vi "校准设置页.vi"() -> ()   [LabVIEW 2016, in "斯坦道通用流路CODmn.lvlib"]
uses:
  <vilib>/regexp/Match Regular Expression.xnode
  <vilib>/ptbypt/NI_PtbyPt.lvlib
panel:
  in  "校准任务":bool
  in  "历史数据导入":T1(radio)
  out "刷新时间":string
  out "模型刷新":bool
  in  "校准按钮":T1(radio)
  in  "仪器写入":bool
  in  "辅助计算":bool
  in  "曲线模型":T2={"标液浓度1"=0.0, "测量吸光度1"=0.0, "样品1启用"=FALSE, "标液浓度2"=0.0, "测量吸光度2"=0.0, "样品2启用"=FALSE, "标液浓度3"=0.0, "测量吸光度3"=0.0, "样品3启用"=FALSE, "标液浓度4"=0.0, "测量吸光度4"=0.0, "样品4启用"=FALSE, "标液浓度5"=0.0, "测量吸光度5"=0.0, "样品5启用"=FALSE, "模型"=enum."线性", "精度"=4.0, "XY图"=[], "拟合公式"="", "r^2"=0.0, "标样一校准时间"=timestamp(0 s since 1904-01-01), "标样二校准时间"=timestamp(0 s since 1904-01-01), "标样三校准时间"=timestamp(0 s since 1904-01-01), "标样四校准时间"=timestamp(0 s since 1904-01-01), "标样五校准时间"=timestamp(0 s since 1904-01-01), "二次方程"={"c"=0.0, "x"=0.0, "x^2"=0.0}, "标定时间"=timestamp(0 s since 1904-01-01)} {"标定时间" format="%<%y/%m/%d %H:%M:%S>T"; "标样五校准时间" format="%<%y/%m/%d %H:%M:%S>T"; "标样四校准时间" format="%<%y/%m/%d %H:%M:%S>T"; "标样三校准时间" format="%<%y/%m/%d %H:%M:%S>T"; "标样二校准时间" format="%<%y/%m/%d %H:%M:%S>T"; "标样一校准时间" format="%<%y/%m/%d %H:%M:%S>T"; "r^2" format="%.7f"; "测量吸光度5" format="%#.6f"; "测量吸光度4" format="%#.6f"; "测量吸光度3" format="%#.6f"; "测量吸光度2" format="%#.6f"; "测量吸光度1" format="%#.6f"}
  in  "测量模式":T3(ring)
  in  "参数下拉列表":u16(ring) items=["氨氮"=3]
  in  "量程下拉列表":enum16{"低量程", "高量程"}(ring)
  # "校准时间"
  # "标液浓度"
  # "吸光值"
  # "标样一"
  # "标样二"
  # "标样三"
  # "零点"
  # "跨度"
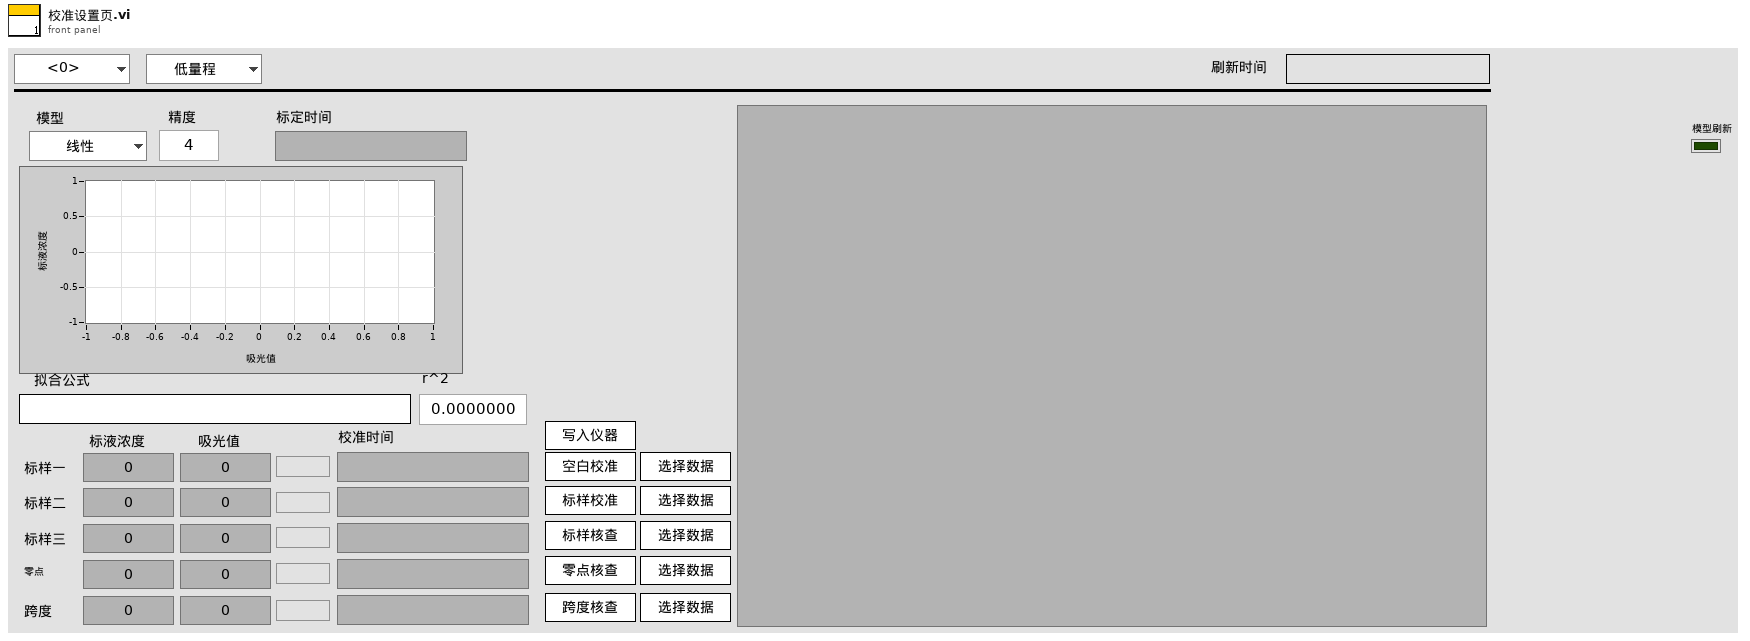
[diagram p1: front panel]
types:
  T1 = enum32{"未选择", "空白校准", "标样校准", "标样核查", "零点核查", "跨度核查"}
  T2 = cluster{"标液浓度1":dbl, "测量吸光度1":dbl, "样品1启用":bool, "标液浓度2":dbl, "测量吸光度2":dbl, "样品2启用":bool, "标液浓度3":dbl, "测量吸光度3":dbl, "样品3启用":bool, "标液浓度4":dbl, "测量吸光度4":dbl, "样品4启用":bool, "标液浓度5":dbl, "测量吸光度5":dbl, "样品5启用":bool, "模型":enum32{"线性", "多项式"}, "精度":dbl, "XY图":cluster{"X Values":dbl[], "Y Values":dbl[]}[], "拟合公式":string, "r^2":dbl, "标样一校准时间":timestamp, "标样二校准时间":timestamp, "标样三校准时间":timestamp, "标样四校准时间":timestamp, "标样五校准时间":timestamp, "二次方程":cluster{"c":dbl, "x":dbl, "x^2":dbl}, "标定时间":timestamp}
  T3 = enum16{"跨度核查", "水样测量", "零点核查", "标样核查", "加标回收", "快捷测试", "空白校准", "标样校准"}
  T4 = typedef "斯坦道通用流路CODmn.lvlib/校准任务.ctl" = cluster{"id":u16, "任务类型":enum16{"未选择", "空白校准", "标样校准", "标样核查", "零点核查", "跨度核查"}, "量程下拉列表":enum16{"低量程", "高量程"}, "状态":enum16{"已执行", "待执行", "执行中", "停止"}, "标液浓度":dbl, "吸光值":dbl, "校准时间":timestamp}
  T5 = enum8{"Enabled", "Disabled", "Disabled and Grayed Out"}
  T6 = cluster{"标液浓度1":dbl, "测量吸光度1":dbl, "样品1启用":bool, "标液浓度2":dbl, "测量吸光度2":dbl, "样品2启用":bool, "标液浓度3":dbl, "测量吸光度3":dbl, "样品3启用":bool, "标液浓度4":dbl, "测量吸光度4":dbl, "样品4启用":bool, "标液浓度5":dbl, "测量吸光度5":dbl, "样品5启用":bool, "模型":enum32{"线性", "多项式"}, "精度":dbl, "XY图":cluster{"X Values":dbl[], "Y Values":dbl[]}[], "拟合公式":string, "r^2":dbl, "标样一校准时间":timestamp, "标样二校准时间":timestamp, "标样三校准时间":timestamp, "标样四校准时间":timestamp, "标样五校准时间":timestamp, "二次方程":cluster{"c":dbl, "x":dbl, "x^2":dbl}, "标定时间":timestamp}[]
  T7 = cluster{"标液浓度1":dbl, "测量吸光度1":dbl, "样品1启用":bool, "标液浓度2":dbl, "测量吸光度2":dbl, "样品2启用":bool, "标液浓度3":dbl, "测量吸光度3":dbl, "样品3启用":bool, "标液浓度4":dbl, "测量吸光度4":dbl, "样品4启用":bool, "标液浓度5":dbl, "测量吸光度5":dbl, "样品5启用":bool, "模型":enum32{"线性", "多项式"}, "精度":dbl, "XY图":cluster{"X Values":dbl[], "Y Values":dbl[]}[], "拟合公式":string, "r^2":dbl, "标样一校准时间":timestamp, "标样二校准时间":timestamp, "标样三校准时间":timestamp, "标样四校准时间":timestamp, "标样五校准时间":timestamp, "二次方程":cluster{"c":dbl, "x":dbl, "x^2":dbl}, "标定时间":timestamp}[][]
  T8 = cluster{"低标液1浓度":dbl, "低标液1信号值":dbl, "低标液1启用":u16, "低标液2浓度":dbl, "低标液2信号值":dbl, "低标液2启用":u16, "低标液3浓度":dbl, "低标液3信号值":dbl, "低标液3启用":u16, "低标液4浓度":dbl, "低标液4信号值":dbl, "低标液4启用":u16, "低标液5浓度":dbl, "低标液5信号值":dbl, "低标液5启用":u16, "高标液1浓度":dbl, "高标液1信号值":dbl, "高标液1启用":u16, "高标液2浓度":dbl, "高标液2信号值":dbl, "高标液2启用":u16, "高标液3浓度":dbl, "高标液3信号值":dbl, "高标液3启用":u16, "高标液4浓度":dbl, "高标液4信号值":dbl, "高标液4启用":u16, "高标液5浓度":dbl, "高标液5信号值":dbl, "高标液5启用":u16, "低斜率":dbl, "低截距":dbl, "低二次多项式系数":dbl, "低线性相关系数":dbl, "高斜率":dbl, "高截距":dbl, "高二次多项式系数":dbl, "高线性相关系数":dbl}
  T9 = typedef "LVStringsAndValuesArrayTypeDef_U16.ctl" = cluster{"String":string, "Value":u16}[]
  T10 = cluster{"系统时间":timestamp, "工作状态":u16, "测量模式":enum16{"待机", "连续模式", "周期模式", "定点模式", "受控模式", "手动模式"}, "告警代码":u16, "故障代码":u16, "日志代码":u16, "软件版本":u16, "F0":sgl, "F1":sgl, "F2":sgl, "F3":sgl, "T":sgl, "H":sgl, "id":u16, "flowid":u16, "量程":u16, "总磷控温温度1":sgl, "营养盐控温温度2":sgl, "ADC":sgl}
  T11 = cluster{"时间":timestamp, "标液值":dbl, "检测值":dbl, "吸光值":dbl}
  T12 = enum32{"Bad", "Idle", "Run top level", "Running"}
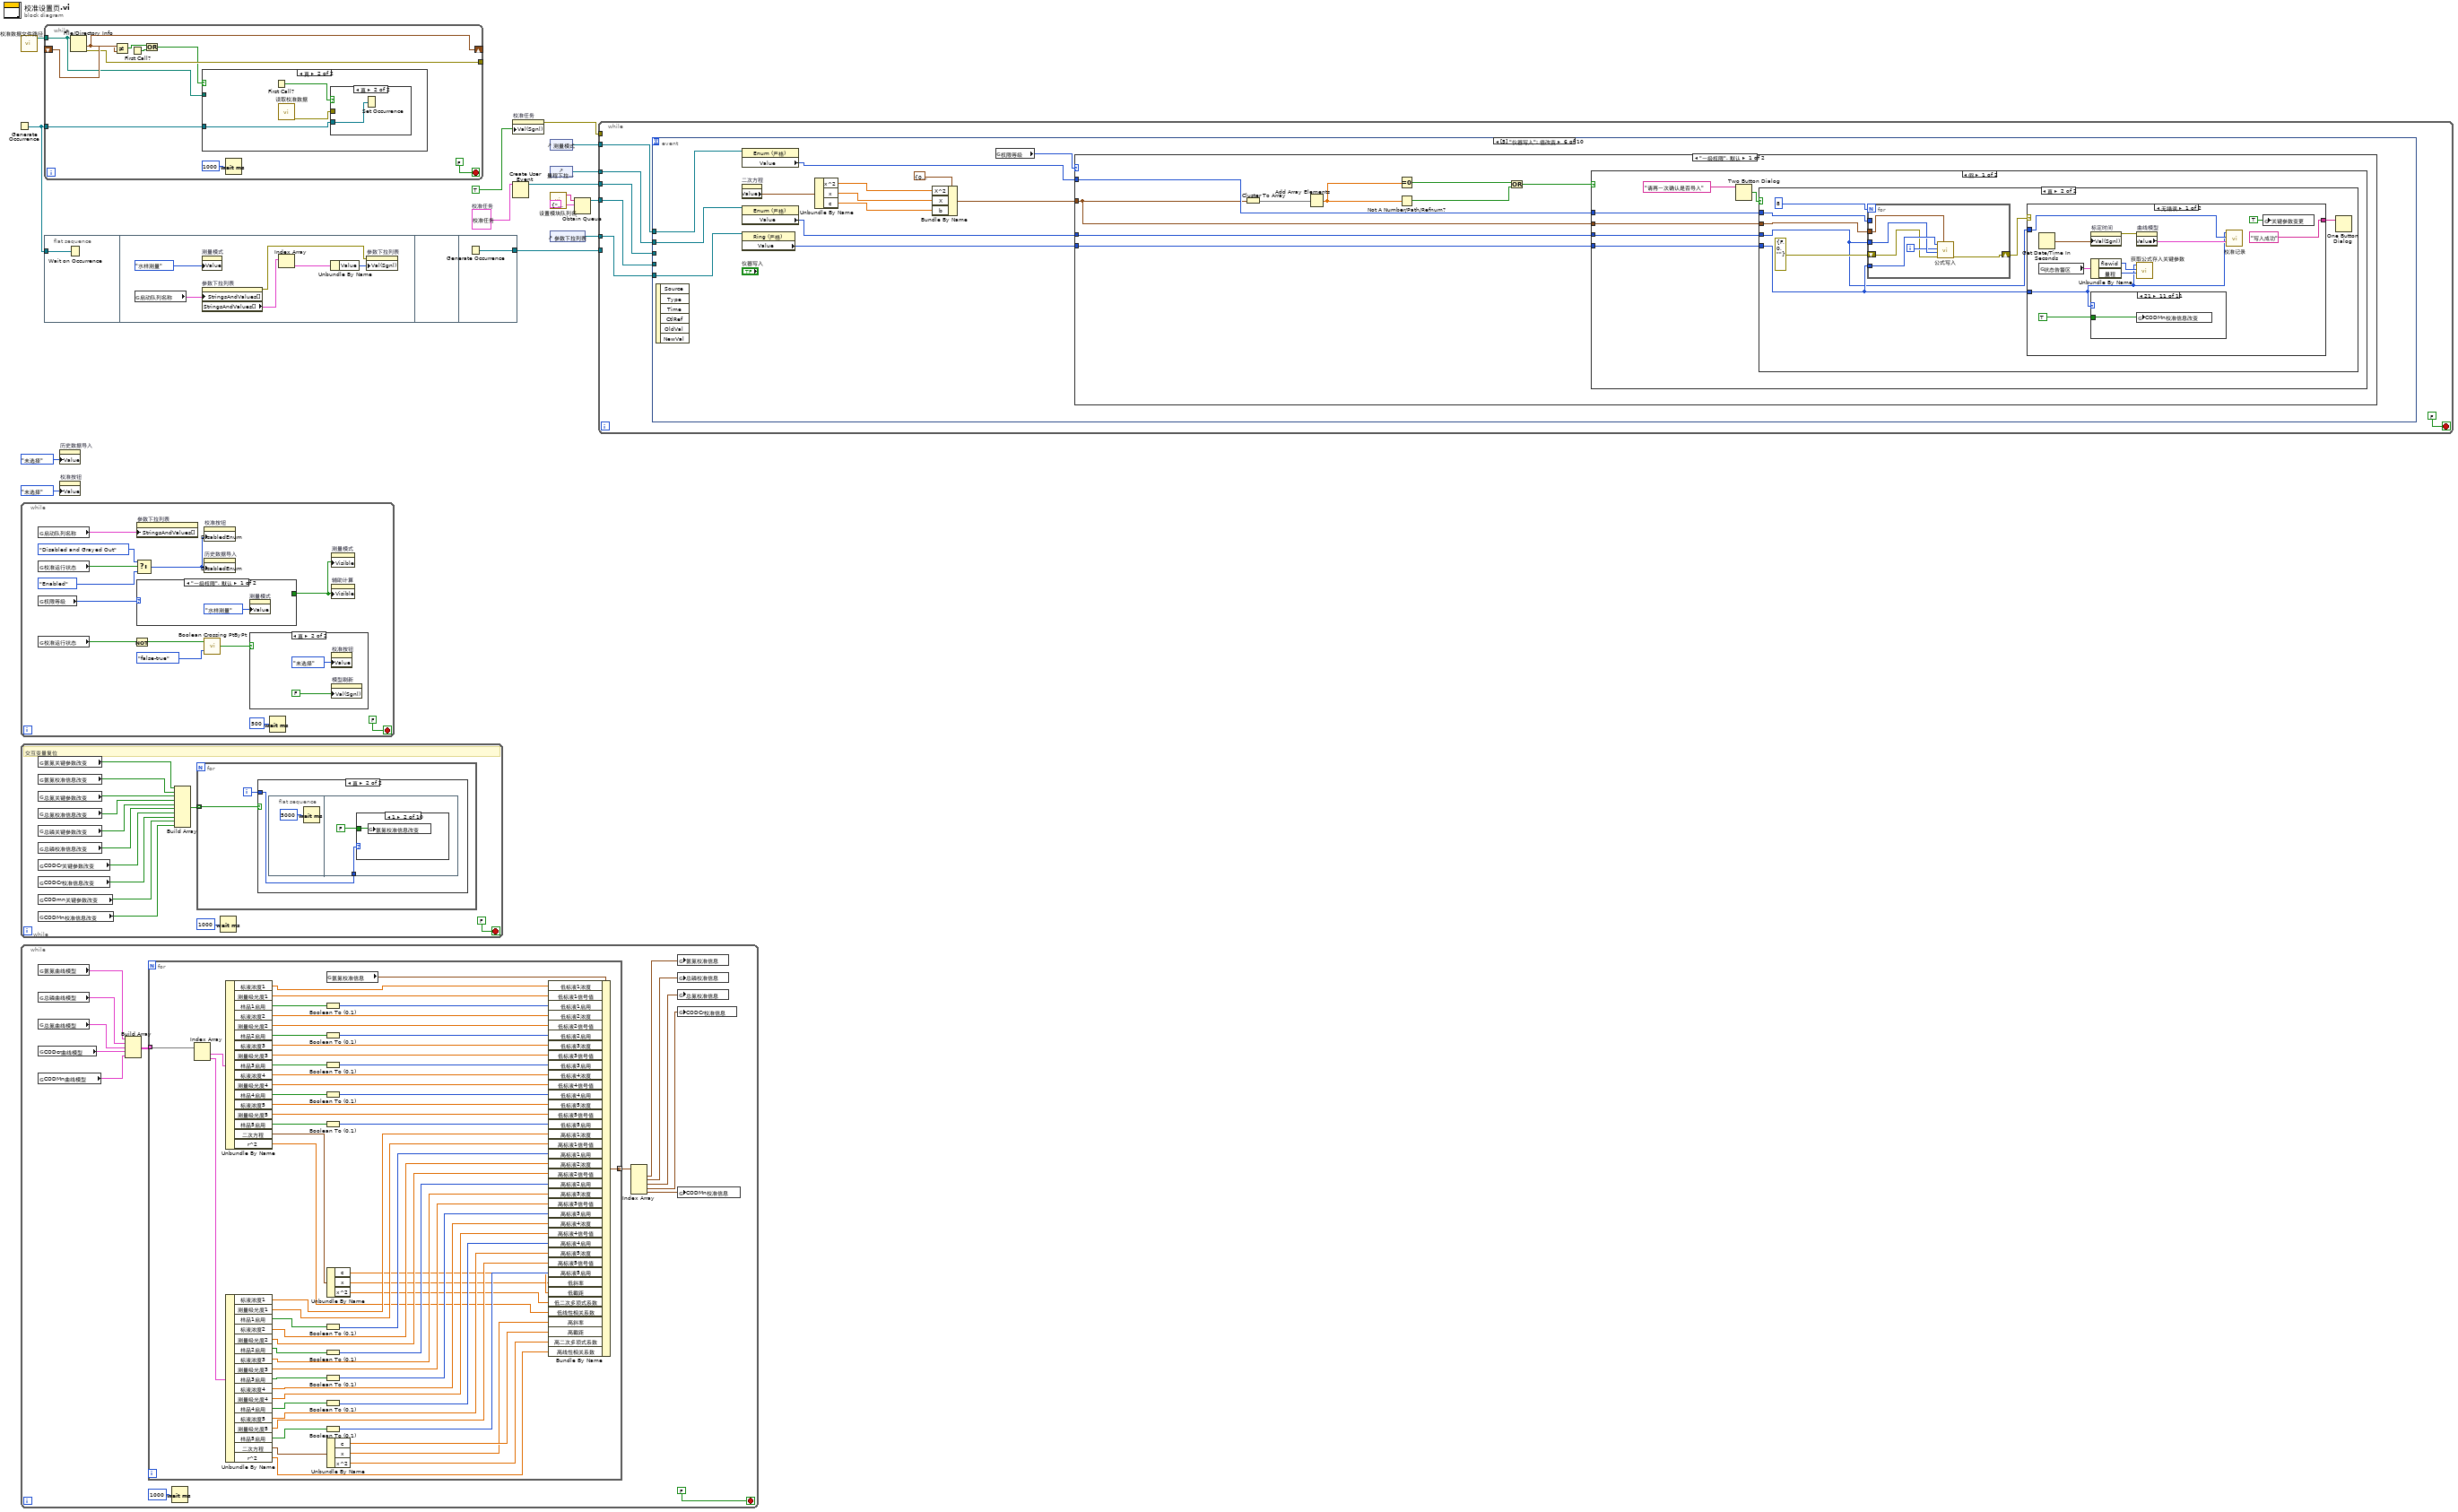
[diagram p0: block diagram]
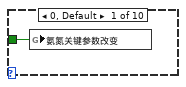
[diagram p3: hidden frame]
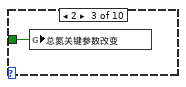
[diagram p4: hidden frame]
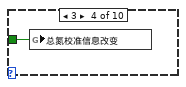
[diagram p5: hidden frame]
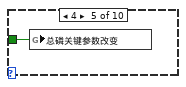
[diagram p6: hidden frame]
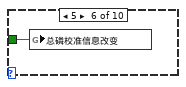
[diagram p7: hidden frame]
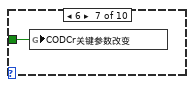
[diagram p8: hidden frame]
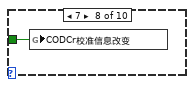
[diagram p9: hidden frame]
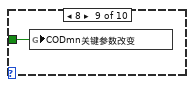
[diagram p10: hidden frame]
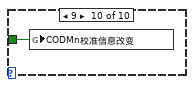
[diagram p11: hidden frame]
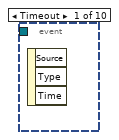
[diagram p14: hidden frame]
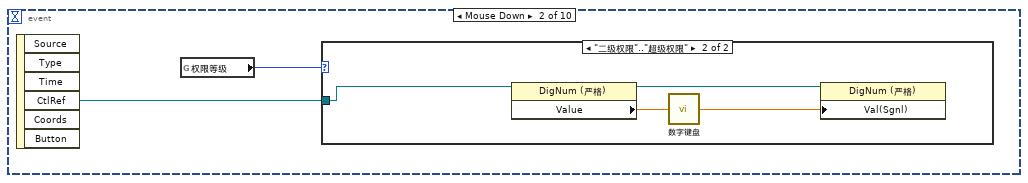
[diagram p15: hidden frame]
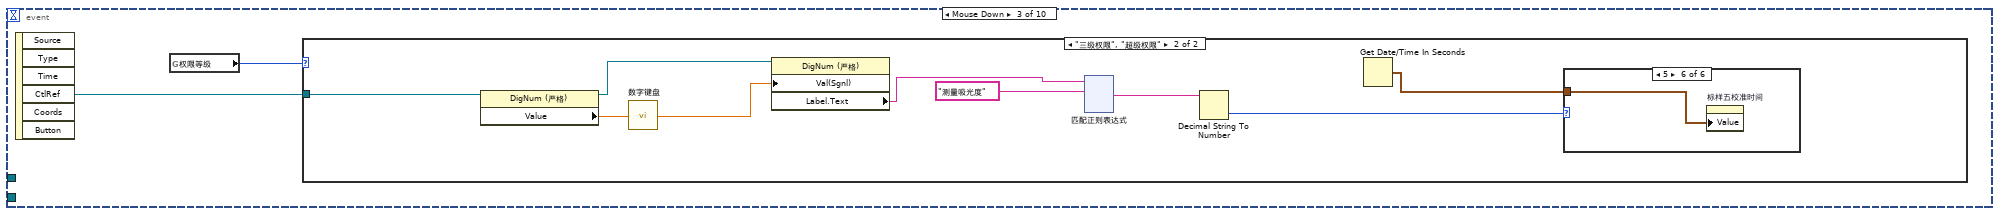
[diagram p17: hidden frame]
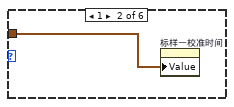
[diagram p20: hidden frame]
diagram:
  w4 = T4 {"id"=1, "任务类型"=enum."未选择", "量程下拉列表"=enum."低量程", "状态"=enum."已执行", "标液浓度"=0.0, "吸光值"=0.0, "校准时间"=timestamp(0 s since 1904-01-01)}  # 校准任务
  n1 = Generate Occurrence() -> (w6:refnum<k4>)
  n2 = call "校准数据文件路径.vi"() -> ("appended path"=w1:path)  [unwired: 11 in]
  n3 = while {
    stop <- FALSE stop-if-true
    n4 = global read "model config var.vi" "启动队列名称"() -> (w23:cluster{"String":string, "Value":u16}[])
    n5 = global read "VAR总磷总氮全局变量.vi" "校准运行状态"() -> (w20:bool)
    n6 = global read "VAR总磷总氮全局变量.vi" "权限等级"() -> (w26:enum16{"一级权限", "二级权限", "三级权限", "超级权限"})
    n7 = global read "VAR总磷总氮全局变量.vi" "校准运行状态"() -> (w22:bool)
    n8 = Not(x=w22) -> (.not. x?=w21:bool)
    n9 = Select(t=T5."Disabled and Grayed Out" ("禁用"), s=w20, f=T5."Enabled" ("禁用")) -> (s? t:f=w18:T5)
    n10 = property on="参数下拉列表" class="Ring (严格)"("StringsAndValues[]"=w23) -> ()  [unwired: 2 in, 2 out]
    n11 = case shown="\"一级权限\", 默认" w26 {
      tunnel: [_ TRUE ("可见")] -> w16
      frame "一级权限", Default {
        n12 = property on="测量模式" class="Enum (严格)"("Value"=T3."水样测量" ("测量模式")) -> ()  [unwired: 2 in, 2 out]
      }
      frame "三级权限", "超级权限" {
      }
    }
    n13 = property on="校准按钮" class="RadioBtnsControl (严格)"("DisabledEnum"=w18) -> ()  [unwired: 2 in, 2 out]
    n14 = property on="历史数据导入" class="RadioBtnsControl (严格)"("DisabledEnum"=w18) -> ()  [unwired: 2 in, 2 out]
    n15 = call <vilib>:"Boolean Crossing PtByPt.vi"("direction"=enum16{"either", "false-true", "true-false"}."false-true", "input"=w21) -> ("crossing"=w24:bool)  [unwired: 1 in]
    n16 = case shown="真" w24 {
      frame False {
      }
      frame True {
        n17 = property on="校准按钮" class="RadioBtnsControl (严格)"("Value"=T1."未选择" ("校准按钮")) -> ()  [unwired: 2 in, 2 out]
        n18 = property on="模型刷新" class="Bool (严格)"("Val(Sgnl)"=FALSE ("值(信号)")) -> ()  [unwired: 2 in, 2 out]
      }
    }
    n19 = Wait (ms)(milliseconds to wait=u32 500 ("等待时间（毫秒）")) -> ()  [unwired: 1 out]
    n20 = property on="测量模式" class="Enum (严格)"("Visible"=w16) -> ()  [unwired: 2 in, 2 out]
    n21 = property on="辅助计算" class="Bool"("Visible"=w16) -> ()  [unwired: 2 in, 2 out]
  }
  n22 = while {
    stop <- FALSE stop-if-true
    # "交互变量复位"
    n23 = global read "VAR总磷总氮全局变量.vi" "氨氮关键参数改变"() -> (w45:bool)
    n24 = global read "VAR总磷总氮全局变量.vi" "氨氮校准信息改变"() -> (w44:bool)
    n25 = global read "VAR总磷总氮全局变量.vi" "总氮关键参数改变"() -> (w43:bool)
    n26 = global read "VAR总磷总氮全局变量.vi" "总氮校准信息改变"() -> (w42:bool)
    n27 = global read "VAR总磷总氮全局变量.vi" "总磷关键参数改变"() -> (w41:bool)
    n28 = global read "VAR总磷总氮全局变量.vi" "总磷校准信息改变"() -> (w40:bool)
    n29 = global read "VAR总磷总氮全局变量.vi" "CODCr关键参数改变"() -> (w39:bool)
    n30 = global read "VAR总磷总氮全局变量.vi" "CODCr校准信息改变"() -> (w38:bool)
    n31 = global read "VAR总磷总氮全局变量.vi" "CODmn关键参数改变"() -> (w34:bool)
    n32 = global read "VAR总磷总氮全局变量.vi" "CODMn校准信息改变"() -> (w33:bool)
    n33 = Build Array(w45, w44, w43, w42, w41, w40, w39, w38, w34, w33) -> (w37:bool[])
    n34 = for {
      tunnel: w37 -> [w47] mode=indexing
      i -> [w46]
      n35 = case shown="真" w47 {
        tunnel: w46 -> [_ w48]
        frame False {
        }
        frame True {
          n36 = flat-sequence {
            tunnel: w48 -> [w51]
            frame #0 {
              n37 = Wait (ms)(milliseconds to wait=u32 5000 ("等待时间（毫秒）")) -> ()  [unwired: 1 out]
            }
            frame #1 {
              n38 = case shown="1" w51 {
                tunnel: FALSE -> [w52 w53 w54 w55 w56 w57 w58 w59 w60 w61]
                frame 0, Default {
                  n39 = global write "VAR总磷总氮全局变量.vi" "氨氮关键参数改变"(w52) -> ()
                }
                frame 1 {
                  n40 = global write "VAR总磷总氮全局变量.vi" "氨氮校准信息改变"(w53) -> ()
                }
                frame 2 {
                  n41 = global write "VAR总磷总氮全局变量.vi" "总氮关键参数改变"(w54) -> ()
                }
                frame 3 {
                  n42 = global write "VAR总磷总氮全局变量.vi" "总氮校准信息改变"(w55) -> ()
                }
                frame 4 {
                  n43 = global write "VAR总磷总氮全局变量.vi" "总磷关键参数改变"(w56) -> ()
                }
                frame 5 {
                  n44 = global write "VAR总磷总氮全局变量.vi" "总磷校准信息改变"(w57) -> ()
                }
                frame 6 {
                  n45 = global write "VAR总磷总氮全局变量.vi" "CODCr关键参数改变"(w58) -> ()
                }
                frame 7 {
                  n46 = global write "VAR总磷总氮全局变量.vi" "CODCr校准信息改变"(w59) -> ()
                }
                frame 8 {
                  n47 = global write "VAR总磷总氮全局变量.vi" "CODmn关键参数改变"(w60) -> ()
                }
                frame 9 {
                  n48 = global write "VAR总磷总氮全局变量.vi" "CODMn校准信息改变"(w61) -> ()
                }
              }
            }
          }
        }
      }
    }
    n49 = Wait (ms)(milliseconds to wait=u32 1000 ("等待时间（毫秒）")) -> ()  [unwired: 1 out]
  }
  n50 = while {
    stop <- FALSE stop-if-true
    n51 = global read "校准数据全局变量.vi" "氨氮曲线模型"() -> (w75:T6)
    n52 = global read "校准数据全局变量.vi" "总磷曲线模型"() -> (w74:T6)
    n53 = global read "校准数据全局变量.vi" "总氮曲线模型"() -> (w73:T6)
    n54 = global read "校准数据全局变量.vi" "CODcr曲线模型"() -> (w72:T6)
    n55 = global read "校准数据全局变量.vi" "CODMn曲线模型"() -> (w63:T6)
    n56 = Build Array(w75, w74, w73, w72, w63) -> (w71:T7)
    n57 = for {
      tunnel: [w130] -> w70 mode=indexing
      tunnel: w71 -> [w87] mode=indexing
      n58 = Index Array(array=w87) -> (element #1=w129:T2, element #2=w126:T2)  [unwired: 2 in]
      n59 = Unbundle By Name(w129) -> ("标液浓度1"=w114:dbl, "测量吸光度1"=w113:dbl, "样品1启用"=w128:bool, "标液浓度2"=w112:dbl, "测量吸光度2"=w111:dbl, "样品2启用"=w123:bool, "标液浓度3"=w93:dbl, "测量吸光度3"=w92:dbl, "样品3启用"=w122:bool, "标液浓度4"=w91:dbl, "测量吸光度4"=w90:dbl, "样品4启用"=w121:bool, "标液浓度5"=w89:dbl, "测量吸光度5"=w88:dbl, "样品5启用"=w120:bool, "二次方程"=w84:cluster{"c":dbl, "x":dbl, "x^2":dbl}, "r^2"=w85:dbl)
      n60 = Unbundle By Name(w126) -> ("标液浓度1"=w125:dbl, "测量吸光度1"=w124:dbl, "样品1启用"=w119:bool, "标液浓度2"=w101:dbl, "测量吸光度2"=w100:dbl, "样品2启用"=w118:bool, "标液浓度3"=w99:dbl, "测量吸光度3"=w98:dbl, "样品3启用"=w117:bool, "标液浓度4"=w97:dbl, "测量吸光度4"=w96:dbl, "样品4启用"=w116:bool, "标液浓度5"=w95:dbl, "测量吸光度5"=w94:dbl, "样品5启用"=w115:bool, "二次方程"=w80:cluster{"c":dbl, "x":dbl, "x^2":dbl}, "r^2"=w76:dbl)
      n61 = Boolean To (0,1)(Boolean=w128) -> (0, 1=w127:i16)
      n62 = Boolean To (0,1)(Boolean=w123) -> (0, 1=w110:i16)
      n63 = Boolean To (0,1)(Boolean=w122) -> (0, 1=w109:i16)
      n64 = Boolean To (0,1)(Boolean=w121) -> (0, 1=w108:i16)
      n65 = Boolean To (0,1)(Boolean=w120) -> (0, 1=w107:i16)
      n66 = Boolean To (0,1)(Boolean=w119) -> (0, 1=w106:i16)
      n67 = Boolean To (0,1)(Boolean=w118) -> (0, 1=w105:i16)
      n68 = Boolean To (0,1)(Boolean=w117) -> (0, 1=w104:i16)
      n69 = Boolean To (0,1)(Boolean=w116) -> (0, 1=w103:i16)
      n70 = Boolean To (0,1)(Boolean=w115) -> (0, 1=w102:i16)
      n71 = global read "VAR总磷总氮全局变量.vi" "氨氮校准信息"() -> (w86:T8)
      n72 = Unbundle By Name(w84) -> ("c"=w83:dbl, "x"=w82:dbl, "x^2"=w81:dbl)
      n73 = Unbundle By Name(w80) -> ("c"=w79:dbl, "x"=w78:dbl, "x^2"=w77:dbl)
      n74 = Bundle By Name(cluster=w86, "低标液1浓度"=w114, "低标液1信号值"=w113, "低标液1启用"=w127, "低标液2浓度"=w112, "低标液2信号值"=w111, "低标液2启用"=w110, "低标液3浓度"=w93, "低标液3信号值"=w92, "低标液3启用"=w109, "低标液4浓度"=w91, "低标液4信号值"=w90, "低标液4启用"=w108, "低标液5浓度"=w89, "低标液5信号值"=w88, "低标液5启用"=w107, "高标液1浓度"=w125, "高标液1信号值"=w124, "高标液1启用"=w106, "高标液2浓度"=w101, "高标液2信号值"=w100, "高标液2启用"=w105, "高标液3浓度"=w99, "高标液3信号值"=w98, "高标液3启用"=w104, "高标液4浓度"=w97, "高标液4信号值"=w96, "高标液4启用"=w103, "高标液5浓度"=w95, "高标液5信号值"=w94, "高标液5启用"=w102, "低斜率"=w82, "低截距"=w83, "低二次多项式系数"=w81, "低线性相关系数"=w85, "高斜率"=w78, "高截距"=w79, "高二次多项式系数"=w77, "高线性相关系数"=w76) -> (w130:T8)
    }
    n75 = Wait (ms)(milliseconds to wait=u32 1000 ("等待时间（毫秒）")) -> ()  [unwired: 1 out]
    n76 = Index Array(array=w70) -> (element #1=w69:T8, element #2=w68:T8, element #3=w67:T8, element #4=w66:T8, element #5=w62:T8)  [unwired: 5 in]
    n77 = global write "VAR总磷总氮全局变量.vi" "氨氮校准信息"(w69) -> ()
    n78 = global write "VAR总磷总氮全局变量.vi" "总磷校准信息"(w68) -> ()
    n79 = global write "VAR总磷总氮全局变量.vi" "总氮校准信息"(w67) -> ()
    n80 = global write "VAR总磷总氮全局变量.vi" "CODCr校准信息"(w66) -> ()
    n81 = global write "VAR总磷总氮全局变量.vi" "CODMn校准信息"(w62) -> ()
  }
  n82 = while {
    shift-right: [w131] -> _
    shift-left: _ -> [w139]
    tunnel: w1 -> [w137]
    tunnel: [w135] -> _
    tunnel: w6 -> [w134]
    stop <- FALSE stop-if-true
    n83 = File/Directory Info(path=w137) -> (last mod=w131:timestamp, error out=w135:errorcluster)  [unwired: 1 in, 5 out]
    n84 = Not Equal?(x=w139, y=w131) -> (x != y?=w138:bool)
    n85 = First Call?() -> (First Call?: T/F=w132:bool)
    n86 = Or(x=w138, y=w132) -> (x .or. y?=w133:bool)
    n87 = case shown="真" w133 {
      tunnel: w137 -> [_ _]
      tunnel: w134 -> [_ w143]
      frame False {
      }
      frame True {
        n88 = First Call?() -> (First Call?: T/F=w141:bool)
        n89 = call "读取校准数据.vi"() -> ("error out"=w142:errorcluster)  [unwired: 11 in]
        n90 = case shown="真" w141 {
          tunnel: w143 -> [_ w144]
          tunnel: w142 -> [_ _]
          frame False {
          }
          frame True {
            n91 = Set Occurrence(w144) -> ()
          }
        }
      }
    }
    n92 = Wait (ms)(milliseconds to wait=u32 1000 ("等待时间（毫秒）")) -> ()  [unwired: 1 out]
  }
  n93 = flat-sequence {
    tunnel: w6 -> [w145]
    tunnel: [w152] -> w15
    frame #0 {
      n94 = Wait on Occurrence(2:w145) -> ()  [unwired: 2 in, 1 out]
    }
    frame #1 {
      n95 = global read "model config var.vi" "启动队列名称"() -> (w147:cluster{"String":string, "Value":u16}[])
      n96 = property on="测量模式" class="Enum (严格)"("Value"=T3."水样测量" ("测量模式")) -> ()  [unwired: 2 in, 2 out]
      n97 = property on="参数下拉列表" class="Ring (严格)"("StringsAndValues[]"=w147) -> (error out=w150:errorcluster, "StringsAndValues[]"=w148:T9)  [unwired: 2 in, 1 out]
      n98 = Index Array(array=w148) -> (element=w149:cluster{"String":string, "Value":u16})  [unwired: 1 in]
      n99 = Unbundle By Name(w149) -> ("Value"=w151:u16)
      n100 = property on="参数下拉列表" class="Ring (严格)"(error in=w150, "Val(Sgnl)"=w151) -> ()  [unwired: 1 in, 2 out]
    }
    frame #2 {
    }
    frame #3 {
      n101 = Generate Occurrence() -> (w152:refnum<k4>)
    }
  }
  n102 = property on="历史数据导入" class="RadioBtnsControl (严格)"("Value"=T1."未选择" ("历史数据导入")) -> ()  [unwired: 2 in, 2 out]
  n103 = property on="校准按钮" class="RadioBtnsControl (严格)"("Value"=T1."未选择" ("校准按钮")) -> ()  [unwired: 2 in, 2 out]
  n104 = property on="校准任务" class="Bool (严格)"("Val(Sgnl)"=TRUE ("值(信号)")) -> (error out=w3:errorcluster)  [unwired: 2 in, 1 out]
  n105 = Create User Event(user event datatype=w4) -> (user event=w5:refnum<user-event>)  [unwired: 1 in, 1 out]
  n106 = control-ref of="测量模式"() -> (w9:refnum<vi>)
  n107 = control-ref of="量程下拉列表"() -> (w8:refnum<vi>)
  n108 = call "设置模块队列名.vi"() -> ("Msg"=w13:string)  [unwired: 5 in]
  n109 = control-ref of="参数下拉列表"() -> (w10:refnum<vi>)
  n110 = Obtain Queue(name (unnamed)=w13, element data type=cluster{"命令":string, "data":variant} {"命令"="", "data"=variant}) -> (queue out=w12:refnum<queue>)  [unwired: 3 in, 2 out]
  n111 = while {
    tunnel: w15 -> [_]
    tunnel: w10 -> [w157]
    tunnel: w9 -> [w156]
    tunnel: w8 -> [w155]
    tunnel: w12 -> [w154]
    tunnel: w5 -> [w153]
    tunnel: w3 -> [_]
    stop <- FALSE stop-if-true
    n112 = event shown="[5] \"仪器写入\": 值改变" {
      selector: _ -> [_ _ _ _ _ _ _ _ _ _]
      dyn-events: _ -> [_ _ _ _ _ _ _ _ _ _]
      timeout: _ -> [_ _ _ _ _ _ _ _ _ _]
      tunnel: w157 -> [_ _ _ w299 _ w360 w415 w477 w505 _]
      tunnel: w156 -> [_ _ _ _ _ w358 _ w472 w500 _]
      tunnel: w155 -> [_ _ _ w297 _ w356 w413 w476 w504 _]
      tunnel: w154 -> [_ _ _ _ _ _ _ w478 w506 _]
      tunnel: w153 -> [_ _ _ _ _ _ _ w471 w499 w528]
      event Timeout {
        n113 = event-data() -> ()  [unwired: 1 in, 3 out]
      }
      event "曲线模型.标液浓度1", "曲线模型.标液浓度2", "曲线模型.标液浓度3", "曲线模型.标液浓度4", "曲线模型.标液浓度5", "曲线模型.精度": Mouse Down {
        n114 = event-data() -> ("CtlRef"=w160:refnum<vi>)  [unwired: 1 in, 5 out]
        n115 = global read "VAR总磷总氮全局变量.vi" "权限等级"() -> (w159:enum16{"一级权限", "二级权限", "三级权限", "超级权限"})
        n116 = case shown="\"二级权限\"..\"超级权限\"" w159 {
          tunnel: w160 -> [_ w164]
          frame "一级权限", Default {
          }
          frame "二级权限".."超级权限" {
            n117 = property class="DigNum (严格)"(reference=w164) -> (reference out=w162:refnum<vi>, "Value"=w163:dbl)  [unwired: 1 in, 1 out]
            n118 = call "数字键盘.vi"("OldNumber"=w163) -> ("NewNumber"=w161:dbl)
            n119 = property class="DigNum (严格)"(reference=w162, "Val(Sgnl)"=w161) -> ()  [unwired: 1 in, 2 out]
          }
        }
      }
      event "曲线模型.测量吸光度1", "曲线模型.测量吸光度2", "曲线模型.测量吸光度3", "曲线模型.测量吸光度4", "曲线模型.测量吸光度5": Mouse Down {
        n120 = event-data() -> ("CtlRef"=w166:refnum<vi>)  [unwired: 1 in, 5 out]
        n121 = global read "VAR总磷总氮全局变量.vi" "权限等级"() -> (w165:enum16{"一级权限", "二级权限", "三级权限", "超级权限"})
        n122 = case shown="\"三级权限\", \"超级权限\"" w165 {
          tunnel: w166 -> [_ w175]
          frame "一级权限", Default {
          }
          frame "三级权限", "超级权限" {
            n123 = property class="DigNum (严格)"(reference=w175) -> (reference out=w173:refnum<vi>, "Value"=w174:dbl)  [unwired: 1 in, 1 out]
            n124 = call "数字键盘.vi"("OldNumber"=w174) -> ("NewNumber"=w172:dbl)
            n125 = property class="DigNum (严格)"(reference=w173, "Val(Sgnl)"=w172) -> ("Label.Text"=w171:string)  [unwired: 1 in, 2 out]
            n126 = xnode "匹配正则表达式"("输入字符串"=w171, "正则表达式"="测量吸光度") -> ("匹配之后"=w169:string)  [unwired: 4 in, 4 out]
            n127 = Decimal String To Number(string=w169) -> (number=w168:i32)  [unwired: 2 in, 1 out]
            n128 = Get Date/Time In Seconds() -> (seconds since 1Jan1904=w167:timestamp)
            n129 = case shown="5" w168 {
              tunnel: w167 -> [_ w176 w177 w178 w179 w180]
              frame 0, Default {
              }
              frame 1 {
                n130 = property on="标样一校准时间" class="AbsTime (严格)"("Value"=w176) -> ()  [unwired: 2 in, 2 out]
              }
              frame 2 {
                n131 = property on="标样二校准时间" class="AbsTime (严格)"("Value"=w177) -> ()  [unwired: 2 in, 2 out]
              }
              frame 3 {
                n132 = property on="标样三校准时间" class="AbsTime (严格)"("Value"=w178) -> ()  [unwired: 2 in, 2 out]
              }
              frame 4 {
                n133 = property on="标样四校准时间" class="AbsTime (严格)"("Value"=w179) -> ()  [unwired: 2 in, 2 out]
              }
              frame 5 {
                n134 = property on="标样五校准时间" class="AbsTime (严格)"("Value"=w180) -> ()  [unwired: 2 in, 2 out]
              }
            }
          }
        }
      }
      event "参数下拉列表", "量程下拉列表", "测量模式", "模型刷新": Value Change {
        n135 = event-data() -> ()  [unwired: 1 in, 6 out]
        n136 = property class="Enum (严格)"(reference=w297) -> ("Value"=w295:enum16{"低量程", "高量程"})  [unwired: 1 in, 2 out]
        n137 = property class="Ring (严格)"(reference=w299) -> ("Value"=w300:u16)  [unwired: 1 in, 2 out]
        n138 = call "id参数转换.vi"("id"=w300) -> ("table输出"=w298:string)  [unwired: 9 in, 1 out]
        n139 = case shown="\"CODMn\"" w298 {
          tunnel: w295 -> [_ w302 w305 w308 w311 w314 w317 w320 w323 w326 w329 w332]
          tunnel: [T2 {"标液浓度1"=0.0, "测量吸光度1"=0.0, "样品1启用"=FALSE, "标液浓度2"=0.0, "测量吸光度2"=0.0, "样品2启用"=FALSE, "标液浓度3"=0.0, "测量吸光度3"=0.0, "样品3启用"=FALSE, "标液浓度4"=0.0, "测量吸光度4"=0.0, "样品4启用"=FALSE, "标液浓度5"=0.0, "测量吸光度5"=0.0, "样品5启用"=FALSE, "模型"=enum."线性", "精度"=0.0, "XY图"=[], "拟合公式"="", "r^2"=0.0, "标样一校准时间"=timestamp(0 s since 1904-01-01), "标样二校准时间"=timestamp(0 s since 1904-01-01), "标样三校准时间"=timestamp(0 s since 1904-01-01), "标样四校准时间"=timestamp(0 s since 1904-01-01), "标样五校准时间"=timestamp(0 s since 1904-01-01), "二次方程"={"c"=0.0, "x"=0.0, "x^2"=0.0}, "标定时间"=timestamp(0 s since 1904-01-01)} ("总磷曲线模型") w303 w306 w309 w312 w315 w318 w321 w324 w327 w330 w333] -> w296
          frame Default {
          }
          frame "总磷" {
            n140 = global read "校准数据全局变量.vi" "总磷曲线模型"() -> (w304:T6)
            n141 = Index Array(array=w304, index=w302) -> (element=w303:T2)
          }
          frame "总氮" {
            n142 = global read "校准数据全局变量.vi" "总氮曲线模型"() -> (w307:T6)
            n143 = Index Array(array=w307, index=w305) -> (element=w306:T2)
          }
          frame "氨氮" {
            n144 = global read "校准数据全局变量.vi" "氨氮曲线模型"() -> (w310:T6)
            n145 = Index Array(array=w310, index=w308) -> (element=w309:T2)
          }
          frame "磷酸盐" {
            n146 = global read "校准数据全局变量.vi" "磷酸盐曲线模型"() -> (w313:T6)
            n147 = Index Array(array=w313, index=w311) -> (element=w312:T2)
          }
          frame "硝氮" {
            n148 = global read "校准数据全局变量.vi" "硝氮曲线模型"() -> (w316:T6)
            n149 = Index Array(array=w316, index=w314) -> (element=w315:T2)
          }
          frame "亚硝氮" {
            n150 = global read "校准数据全局变量.vi" "亚硝氮曲线模型"() -> (w319:T6)
            n151 = Index Array(array=w319, index=w317) -> (element=w318:T2)
          }
          frame "硅酸盐" {
            n152 = global read "校准数据全局变量.vi" "硅酸盐曲线模型"() -> (w322:T6)
            n153 = Index Array(array=w322, index=w320) -> (element=w321:T2)
          }
          frame "硫化物" {
            n154 = global read "校准数据全局变量.vi" "硫化物曲线模型"() -> (w325:T6)
            n155 = Index Array(array=w325, index=w323) -> (element=w324:T2)
          }
          frame "CODcr" {
            n156 = global read "校准数据全局变量.vi" "CODcr曲线模型"() -> (w328:T6)
            n157 = Index Array(array=w328, index=w326) -> (element=w327:T2)
          }
          frame "CODMn" {
            n158 = global read "校准数据全局变量.vi" "CODMn曲线模型"() -> (w331:T6)
            n159 = Index Array(array=w331, index=w329) -> (element=w330:T2)
          }
          frame "氟化物" {
            n160 = global read "校准数据全局变量.vi" "氟化物曲线模型"() -> (w334:T6)
            n161 = Index Array(array=w334, index=w332) -> (element=w333:T2)
          }
        }
        n162 = property on="曲线模型" class="Clust (严格)"("Val(Sgnl)"=w296) -> ()  [unwired: 2 in, 2 out]
      }
      event "辅助计算": Value Change {
        n163 = event-data() -> ()  [unwired: 1 in, 6 out]
        n164 = Get Date/Time In Seconds() -> (seconds since 1Jan1904=w335:timestamp)
        n165 = call "吸光值辅助计算.vi"() -> ("X"=w336:dbl, "吸光值导出"=w337:u16)  [unwired: 10 in]
        n166 = case shown="4" w337 {
          tunnel: w336 -> [_ w339 w341 w343 w345 w347]
          tunnel: w335 -> [_ w338 w340 w342 w344 w346]
          frame 0, Default {
          }
          frame 1 {
            n167 = property on="标样一校准时间" class="AbsTime (严格)"("Val(Sgnl)"=w338) -> ()  [unwired: 2 in, 2 out]
            n168 = property on="测量吸光度1" class="DigNum (严格)"("Value"=w339) -> ()  [unwired: 2 in, 2 out]
          }
          frame 2 {
            n169 = property on="标样二校准时间" class="AbsTime (严格)"("Val(Sgnl)"=w340) -> ()  [unwired: 2 in, 2 out]
            n170 = property on="测量吸光度2" class="DigNum (严格)"("Value"=w341) -> ()  [unwired: 2 in, 2 out]
          }
          frame 3 {
            n171 = property on="标样三校准时间" class="AbsTime (严格)"("Val(Sgnl)"=w342) -> ()  [unwired: 2 in, 2 out]
            n172 = property on="测量吸光度3" class="DigNum (严格)"("Value"=w343) -> ()  [unwired: 2 in, 2 out]
          }
          frame 4 {
            n173 = property on="标样四校准时间" class="AbsTime (严格)"("Val(Sgnl)"=w344) -> ()  [unwired: 2 in, 2 out]
            n174 = property on="测量吸光度4" class="DigNum (严格)"("Value"=w345) -> ()  [unwired: 2 in, 2 out]
          }
          frame 5 {
            n175 = property on="标样五校准时间" class="AbsTime (严格)"("Val(Sgnl)"=w346) -> ()  [unwired: 2 in, 2 out]
            n176 = property on="测量吸光度5" class="DigNum (严格)"("Value"=w347) -> ()  [unwired: 2 in, 2 out]
          }
        }
      }
      event "仪器写入": Value Change {
        n177 = event-data() -> ()  [unwired: 1 in, 6 out]
        n178 = property class="Enum (严格)"(reference=w358) -> ("Value"=w357:T3)  [unwired: 1 in, 2 out]
        n179 = property on="二次方程" class="Clust (严格)"() -> ("Value"=w349:cluster{"c":dbl, "x":dbl, "x^2":dbl})  [unwired: 2 in, 2 out]
        n180 = property class="Enum (严格)"(reference=w356) -> ("Value"=w355:enum16{"低量程", "高量程"})  [unwired: 1 in, 2 out]
        n181 = property class="Ring (严格)"(reference=w360) -> ("Value"=w359:u16)  [unwired: 1 in, 2 out]
        n182 = Unbundle By Name(w349) -> ("x^2"=w351:dbl, "x"=w352:dbl, "c"=w353:dbl)
        n183 = Bundle By Name(cluster=cluster{"X^2":dbl, "X":dbl, "b":dbl} {"X^2"=0.0, "X"=0.0, "b"=0.0} ("公式"), "X^2"=w351, "X"=w352, "b"=w353) -> (w348:cluster{"X^2":dbl, "X":dbl, "b":dbl})
        n184 = global read "VAR总磷总氮全局变量.vi" "权限等级"() -> (w354:enum16{"一级权限", "二级权限", "三级权限", "超级权限"})
        n185 = case shown="\"一级权限\", 默认" w354 {
          tunnel: w359 -> [w369 w411]
          tunnel: w357 -> [w368 w410]
          tunnel: w355 -> [w367 w409]
          tunnel: w348 -> [w361 w408]
          frame "一级权限", Default {
            n186 = Cluster To Array(cluster=w361) -> (array=w366:dbl[])
            n187 = Add Array Elements(numeric array=w366) -> (sum=w365:dbl)
            n188 = Equal To 0?(x=w365) -> (x = 0?=w363:bool)
            n189 = Not A Number/Path/Refnum?(number/path/refnum=w365) -> (NaN/Path/Refnum?=w364:bool)
            n190 = Or(x=w363, y=w364) -> (x .or. y?=w362:bool)
            n191 = case shown="假" w362 {
              tunnel: w369 -> [w375 _]
              tunnel: w368 -> [w374 _]
              tunnel: w367 -> [w373 _]
              tunnel: w361 -> [w370 _]
              frame False {
                n192 = Two Button Dialog(message="请再一次确认是否导入" ("消息")) -> (T button?=w371:bool)  [unwired: 2 in]
                n193 = case shown="真" w371 {
                  tunnel: w375 -> [_ w377]
                  tunnel: w374 -> [_ w383]
                  tunnel: w373 -> [_ w376]
                  tunnel: w370 -> [_ w378]
                  frame False {
                  }
                  frame True {
                    n194 = for {
                      N: 8 -> [_]
                      tunnel: w377 -> [w389]
                      tunnel: w383 -> [_]
                      tunnel: w376 -> [w388]
                      shift-right: [w387] -> w381
                      shift-left: errorcluster {"status"=FALSE, "code"=0, "source"=""} ("error out") -> [w384]
                      tunnel: w378 -> [w385]
                      i -> [w386]
                      n195 = call "公式写入.vi"("公式"=w385, "error in (no error)"=w384, "量程"=w388, "测量模式"=w386, "测量参数"=w389) -> ("error out"=w387:errorcluster)  [unwired: 6 in]
                    }
                    n196 = case shown="无错误" w381 {
                      tunnel: ["写入成功" "写入失败"] -> w382
                      tunnel: w377 -> [w390 _]
                      tunnel: w376 -> [w398 _]
                      frame No Error {
                        n197 = Get Date/Time In Seconds() -> (seconds since 1Jan1904=w399:timestamp)
                        n198 = global read "VAR总磷总氮全局变量.vi" "状态告警区"() -> (w395:T10)
                        n199 = property on="标定时间" class="AbsTime (严格)"("Val(Sgnl)"=w399) -> (error out=w396:errorcluster)  [unwired: 2 in, 1 out]
                        n200 = Unbundle By Name(w395) -> ("flowid"=w393:u16, "量程"=w394:u16)
                        n201 = case shown="21" w390 {
                          tunnel: TRUE ("总磷关键参数改变") -> [_ w401 w402 w403 _ _ _ _ _ w404 w405]
                          frame 0, Default {
                          }
                          frame 1 {
                            n202 = global write "VAR总磷总氮全局变量.vi" "总磷校准信息改变"(w401) -> ()
                          }
                          frame 2 {
                            n203 = global write "VAR总磷总氮全局变量.vi" "总氮校准信息改变"(w402) -> ()
                          }
                          frame 3 {
                            n204 = global write "VAR总磷总氮全局变量.vi" "氨氮校准信息改变"(w403) -> ()
                          }
                          frame 4 {
                          }
                          frame 5 {
                          }
                          frame 6 {
                          }
                          frame 7 {
                          }
                          frame 8 {
                          }
                          frame 22 {
                            n205 = global write "VAR总磷总氮全局变量.vi" "CODCr校准信息改变"(w404) -> ()
                          }
                          frame 21 {
                            n206 = global write "VAR总磷总氮全局变量.vi" "CODMn校准信息改变"(w405) -> ()
                          }
                        }
                        n207 = property on="曲线模型" class="Clust (严格)"(error in=w396) -> ("Value"=w397:T2)  [unwired: 1 in, 2 out]
                        n208 = call "获取公式存入关键参数.vi"("量程"=w394, "flowid"=w393, "id"=w390) -> ()  [unwired: 7 in, 2 out]
                        n209 = call "校准记录.vi"("曲线模型"=w397, "量程"=w398, "校准参数"=w390) -> ()  [unwired: 8 in, 1 out]
                        n210 = global write "VAR总磷总氮全局变量.vi" "关键参数变更"(TRUE ("关键参数变更")) -> ()
                      }
                      frame Error {
                      }
                    }
                    n211 = One Button Dialog(message=w382) -> ()  [unwired: 1 in, 1 out]
                  }
                }
              }
              frame True {
                n212 = One Button Dialog(message="校准数据异常，请重新校准！" ("消息")) -> ()  [unwired: 1 in, 1 out]
              }
            }
          }
          frame "三级权限", "超级权限" {
            n213 = call "公式复合写入.vi"("公式"=w408, "量程下拉列表"=w409, "测量模式"=w410, "参数下拉列表"=w411) -> ()  [unwired: 8 in]
          }
        }
      }
      event "曲线模型": Value Change {
        n214 = event-data() -> ()  [unwired: 1 in, 6 out]
        n215 = flat-sequence {
          tunnel: [w420] -> w416
          tunnel: w415 -> [w420]
          tunnel: [w419] -> w414
          tunnel: w413 -> [w419]
          tunnel: w416 -> [w426]
          tunnel: w414 -> [w423]
          frame #0 {
            n216 = property on="曲线模型" class="Clust (严格)"() -> ("Value"=w418:T2)  [unwired: 2 in, 2 out]
            n217 = call "曲线模型计算.vi"("曲线模型"=w418) -> ("输出簇"=w417:T2)  [unwired: 10 in]
            n218 = property on="曲线模型" class="Clust (严格)"("Value"=w417) -> ()  [unwired: 2 in, 2 out]
          }
          frame #1 {
            n219 = property class="Enum (严格)"(reference=w423) -> ("Value"=w422:enum16{"低量程", "高量程"})  [unwired: 1 in, 2 out]
            n220 = property class="Ring (严格)"(reference=w426) -> ("Value"=w425:u16)  [unwired: 1 in, 2 out]
            n221 = call "id参数转换.vi"("id"=w425) -> ("table输出"=w424:string)  [unwired: 9 in, 1 out]
            n222 = property on="曲线模型" class="Clust (严格)"() -> ("Value"=w421:T2)  [unwired: 2 in, 2 out]
            n223 = case shown="\"CODcr\"" w424 {
              tunnel: w421 -> [_ w428 w434 w437 w440 w444 w448 w452 w456 w461 w465 w469]
              tunnel: w422 -> [_ w427 w431 w435 w439 w443 w447 w451 w455 w459 w463 w467]
              frame Default {
              }
              frame "总磷" {
                n224 = global read "校准数据全局变量.vi" "总磷曲线模型"() -> (w429:T6)
                n225 = Replace Array Subset(array=w429, new element=w428, index=w427) -> (w430:T6)
                n226 = global write "校准数据全局变量.vi" "总磷曲线模型"(w430) -> ()
              }
              frame "总氮" {
                n227 = global read "校准数据全局变量.vi" "总氮曲线模型"() -> (w433:T6)
                n228 = Replace Array Subset(array=w433, new element=w434, index=w431) -> (w432:T6)
                n229 = global write "校准数据全局变量.vi" "总氮曲线模型"(w432) -> ()
              }
              frame "氨氮" {
                n230 = global read "校准数据全局变量.vi" "氨氮曲线模型"() -> (w438:T6)
                n231 = Replace Array Subset(array=w438, new element=w437, index=w435) -> (w436:T6)
                n232 = global write "校准数据全局变量.vi" "氨氮曲线模型"(w436) -> ()
              }
              frame "磷酸盐" {
                n233 = global read "校准数据全局变量.vi" "磷酸盐曲线模型"() -> (w442:T6)
                n234 = Replace Array Subset(array=w442, new element=w440, index=w439) -> (w441:T6)
                n235 = global write "校准数据全局变量.vi" "磷酸盐曲线模型"(w441) -> ()
              }
              frame "硝氮" {
                n236 = global read "校准数据全局变量.vi" "硝氮曲线模型"() -> (w446:T6)
                n237 = Replace Array Subset(array=w446, new element=w444, index=w443) -> (w445:T6)
                n238 = global write "校准数据全局变量.vi" "硝氮曲线模型"(w445) -> ()
              }
              frame "亚硝氮" {
                n239 = global read "校准数据全局变量.vi" "亚硝氮曲线模型"() -> (w450:T6)
                n240 = Replace Array Subset(array=w450, new element=w448, index=w447) -> (w449:T6)
                n241 = global write "校准数据全局变量.vi" "亚硝氮曲线模型"(w449) -> ()
              }
              frame "硅酸盐" {
                n242 = global read "校准数据全局变量.vi" "硅酸盐曲线模型"() -> (w454:T6)
                n243 = Replace Array Subset(array=w454, new element=w452, index=w451) -> (w453:T6)
                n244 = global write "校准数据全局变量.vi" "硅酸盐曲线模型"(w453) -> ()
              }
              frame "硫化物" {
                n245 = global read "校准数据全局变量.vi" "硫化物曲线模型"() -> (w458:T6)
                n246 = Replace Array Subset(array=w458, new element=w456, index=w455) -> (w457:T6)
                n247 = global write "校准数据全局变量.vi" "硫化物曲线模型"(w457) -> ()
              }
              frame "CODcr" {
                n248 = global read "校准数据全局变量.vi" "CODcr曲线模型"() -> (w462:T6)
                n249 = Replace Array Subset(array=w462, new element=w461, index=w459) -> (w460:T6)
                n250 = global write "校准数据全局变量.vi" "CODcr曲线模型"(w460) -> ()
              }
              frame "CODMn" {
                n251 = global read "校准数据全局变量.vi" "CODMn曲线模型"() -> (w466:T6)
                n252 = Replace Array Subset(array=w466, new element=w465, index=w463) -> (w464:T6)
                n253 = global write "校准数据全局变量.vi" "CODMn曲线模型"(w464) -> ()
              }
              frame "氟化物" {
                n254 = global read "校准数据全局变量.vi" "氟化物曲线模型"() -> (w470:T6)
                n255 = Replace Array Subset(array=w470, new element=w469, index=w467) -> (w468:T6)
                n256 = global write "校准数据全局变量.vi" "氟化物曲线模型"(w468) -> ()
              }
            }
          }
          frame #2 {
            n257 = call "校准数据写入配置文件.vi"() -> ()  [unwired: 11 in, 1 out]
          }
        }
        n258 = Format Date/Time String() -> (date/time string=→"刷新时间":string)  [unwired: 3 in]
      }
      event "校准按钮": Value Change {
        n259 = event-data() -> ("NewVal"=w473:T1)  [unwired: 1 in, 5 out]
        n260 = Not Equal?(x=w473, y=T1."未选择") -> (x != y?=w474:bool)
        n261 = case shown="真" w474 {
          tunnel: w478 -> [_ _]
          tunnel: w477 -> [_ w488]
          tunnel: w476 -> [_ w487]
          tunnel: w473 -> [_ w483]
          tunnel: w472 -> [_ _]
          tunnel: w471 -> [_ w486]
          frame False {
          }
          frame True {
            w480 = T4 {"id"=1, "任务类型"=enum."未选择", "量程下拉列表"=enum."低量程", "状态"=enum."待执行", "标液浓度"=0.0, "吸光值"=0.0, "校准时间"=timestamp(0 s since 1904-01-01)}  # 校准任务
            n262 = property class="Enum (严格)"(reference=w487) -> ("Value"=w484:enum16{"低量程", "高量程"})  [unwired: 1 in, 2 out]
            n263 = property on="曲线模型" class="Clust (严格)"() -> ("Value"=w482:T2)  [unwired: 2 in, 2 out]
            n264 = property class="Ring (严格)"(reference=w488) -> ("Value"=w485:u16)  [unwired: 1 in, 2 out]
            n265 = case shown="\"未选择\", 默认" w483 {
              tunnel: w482 -> [_ w490 w492 w494 w496 w498]
              tunnel: [_ w489 w491 w493 w495 w497] -> w481
              frame "未选择", Default {
              }
              frame "空白校准" {
                n266 = Unbundle By Name(w490) -> ("标液浓度1"=w489:dbl)
              }
              frame "标样校准" {
                n267 = Unbundle By Name(w492) -> ("标液浓度2"=w491:dbl)
              }
              frame "标样核查" {
                n268 = Unbundle By Name(w494) -> ("标液浓度3"=w493:dbl)
              }
              frame "零点核查" {
                n269 = Unbundle By Name(w496) -> ("标液浓度4"=w495:dbl)
              }
              frame "跨度核查" {
                n270 = Unbundle By Name(w498) -> ("标液浓度5"=w497:dbl)
              }
            }
            n271 = Bundle By Name(cluster=w480, "id"=w485, "任务类型"=w483, "量程下拉列表"=w484, "标液浓度"=w481) -> (w479:T4)
            n272 = Generate User Event(user event=w486, event data cluster=w479) -> ()  [unwired: 2 in, 2 out]
          }
        }
      }
      event "历史数据导入": Value Change {
        n273 = event-data() -> ("NewVal"=w501:T1)  [unwired: 1 in, 5 out]
        n274 = Not Equal?(x=w501, y=T1."未选择") -> (x != y?=w502:bool)
        n275 = case shown="真" w502 {
          tunnel: w506 -> [_ _]
          tunnel: w505 -> [_ w516]
          tunnel: w504 -> [_ w509]
          tunnel: w501 -> [_ w507]
          tunnel: w500 -> [_ _]
          tunnel: w499 -> [_ w511]
          frame False {
          }
          frame True {
            n276 = property class="Enum (严格)"(reference=w509) -> ("Value"=w508:enum16{"低量程", "高量程"})  [unwired: 1 in, 2 out]
            n277 = property class="Ring (严格)"(reference=w516) -> ("Value"=w510:u16)  [unwired: 1 in, 2 out]
            n278 = property on="历史数据导入" class="RadioBtnsControl (严格)"("Value"=T1."未选择" ("历史数据导入")) -> ()  [unwired: 2 in, 2 out]
            n279 = call "id参数转换.vi"("id"=w510) -> ("table输出"=w515:string)  [unwired: 9 in, 1 out]
            n280 = call "校准数据选择表.vi"("测量模式"=w507, "量程下拉列表"=w508, "table"=w515) -> ("布尔"=w514:bool, "输出"=w513:T11)  [unwired: 7 in]
            n281 = case shown="真" w514 {
              tunnel: w513 -> [_ w524]
              tunnel: w507 -> [_ w526]
              tunnel: w511 -> [_ w525]
              tunnel: w510 -> [_ w523]
              tunnel: w508 -> [_ w522]
              frame False {
              }
              frame True {
                w520 = T4 {"id"=1, "任务类型"=enum."未选择", "量程下拉列表"=enum."低量程", "状态"=enum."已执行", "标液浓度"=0.0, "吸光值"=0.0, "校准时间"=timestamp(0 s since 1904-01-01)}  # 校准任务
                n282 = Unbundle By Name(w524) -> ("标液值"=w517:dbl, "吸光值"=w518:dbl, "时间"=w519:timestamp)
                n283 = Bundle By Name(cluster=w520, "id"=w523, "任务类型"=w526, "量程下拉列表"=w522, "标液浓度"=w517, "吸光值"=w518, "校准时间"=w519) -> (w521:T4)
                n284 = Generate User Event(user event=w525, event data cluster=w521) -> ()  [unwired: 2 in, 2 out]
              }
            }
          }
        }
      }
      event "校准任务": Value Change {
        n285 = event-data() -> ("NewVal"=w527:bool)  [unwired: 1 in, 5 out]
        n286 = invoke on="子面板" class="SubPnl" method="Remove VI"() -> (error out=w529:errorcluster)  [unwired: 3 in, 2 out]
        n287 = case shown="真" w527 {
          tunnel: w529 -> [_ w536]
          tunnel: w528 -> [_ w533]
          frame False {
          }
          frame True {
            n288 = vi-ref "校准任务设置.vi"() -> (w535:refnum<vi>)
            n289 = property class="VI"(reference=w535) -> (reference out=w531:refnum<vi>, "Name"=w534:string, "Exec.State"=w532:T12)  [unwired: 1 in, 1 out]
            n290 = case shown="\"Idle\"" w532 {
              tunnel: w534 -> [_ w548]
              tunnel: w533 -> [_ w545]
              tunnel: [w537 w541] -> w530
              tunnel: w531 -> [w537 w541]
              frame "Bad", Default {
              }
              frame "Idle" {
                n291 = Open VI Reference(type specifier VI Refnum (for type only)=refnum<vi> refnum, vi path=w548, options=128 ("选项")) -> (vi reference=w546:refnum<vi>, error out=w543:errorcluster)  [unwired: 3 in]
                n292 = property on="模型" class="Enum (严格)"() -> ("Value"=w539:enum32{"线性", "多项式"})  [unwired: 2 in, 2 out]
                n293 = property on="精度" class="DigNum (严格)"() -> ("Value"=w538:dbl)  [unwired: 2 in, 2 out]
                n294 = call-by-ref "开始异步调用"(reference=w546, error in=w543, "精度"=w538, "模型"=w539, "用户事件"=w545) -> (reference out=w544:refnum<vi>, error out=w542:errorcluster)  [unwired: 9 in]
                n295 = Close Reference(reference=w544, error in (no error)=w542) -> ()  [unwired: 1 out]
              }
            }
            n296 = invoke on="子面板" class="SubPnl" method="Insert VI"(error in=w536, "VI Ref"=w530) -> ()  [unwired: 2 in, 4 out]
          }
        }
      }
    }
  }
